vi "Map Grap to Chart.vi"(11 "CVM":cluster{i32[], dbl[]}[](graph)) -> (3 "Cell Voltages":waveform(dbl)[](graph))   [LabVIEW 2025, in "Controller_TV_STK_01.lvlib"]
uses:
  labview-tv-stk-01/Libraries/Controller_TV_STK_01/Controller_TV_STK_01.lvlib
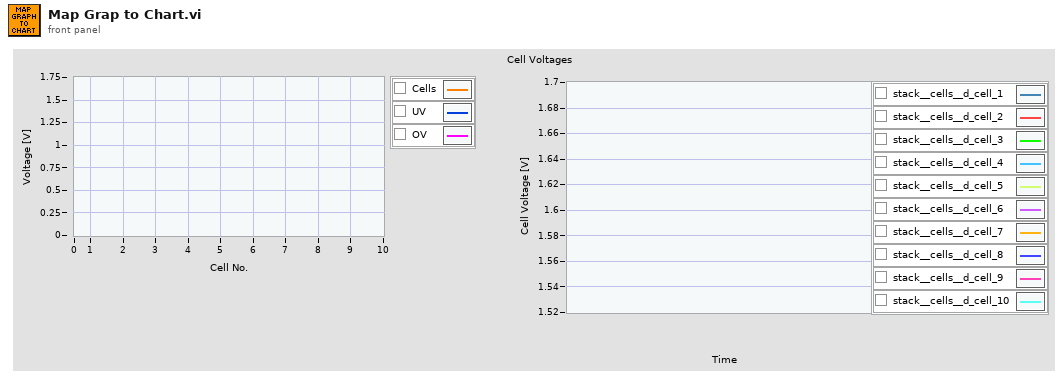
[diagram p1: front panel]
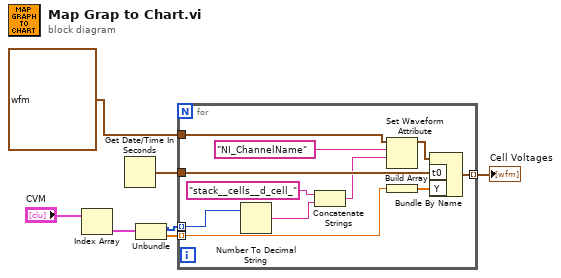
[diagram p0: block diagram]
diagram:
  n1 = Index Array(array="CVM") -> (element=w6:cluster{i32[], dbl[]})  [unwired: 1 in]
  n2 = Get Date/Time In Seconds() -> (seconds since 1Jan1904=w2:timestamp)
  n3 = Unbundle(w6) -> (w1:i32[], w4:dbl[])
  n4 = for {
    tunnel: w2 -> [w18]
    tunnel: [w16] -> w5 mode=indexing
    tunnel: waveform(dbl) {"t0"=timestamp(0 s since 1904-01-01), "dt"=1.0, "Y"=[]} ("waveform") -> [w15]
    tunnel: w4 -> [w12] mode=indexing
    tunnel: w1 -> [w11] mode=indexing
    n5 = Number To Decimal String(number=w11) -> (decimal integer string=w9:string)  [unwired: 1 in]
    n6 = Concatenate Strings("stack__cells__d_cell_", w9) -> (w8:string)
    n7 = Set Waveform Attribute(5:w8, 6:"NI_ChannelName" ("name"), 7:w15) -> (3:w17:waveform(dbl))  [unwired: 1 in, 2 out]
    n8 = Build Array(w12) -> (w14:dbl[])
    n9 = Bundle By Name(cluster=w17, "t0"=w18, "Y"=w14) -> (w16:waveform(dbl))
  }
  "Cell Voltages" <- w5
